vi "加减乘除运算.vi"(1 "符号":string[](array[string]), 2 "元素":string[](array[string])) -> (0 "结果":string)   [LabVIEW 2014]
panel:
  out "输出符号":string[](array[string])
  out "输出元素":string[](array[string])
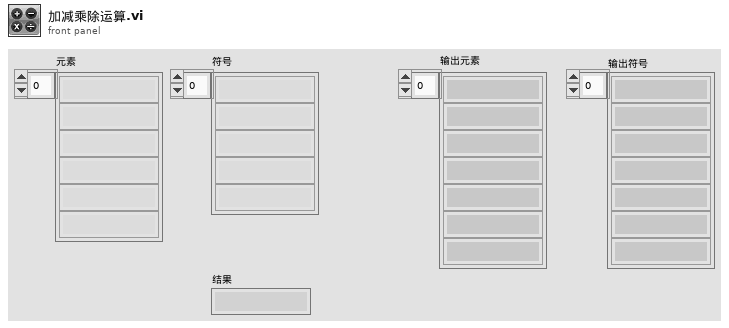
[diagram p1: front panel]
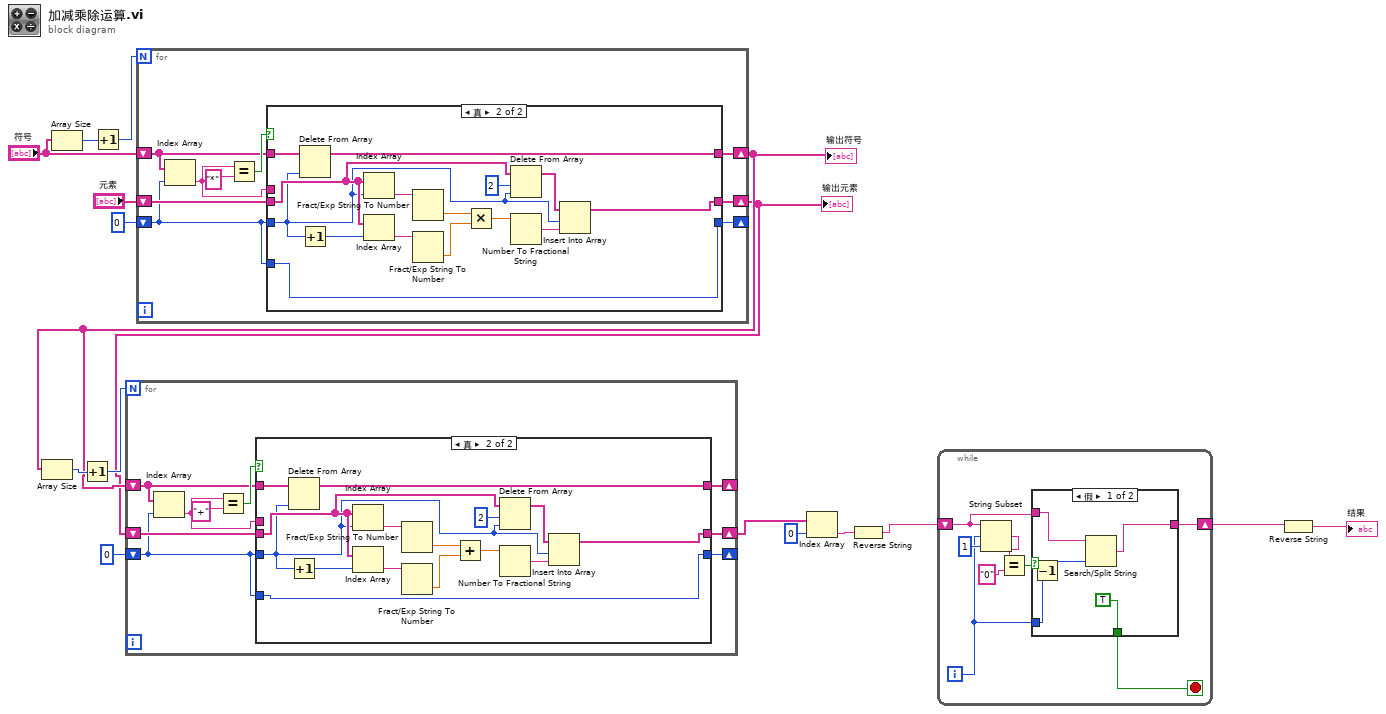
[diagram p0: block diagram]
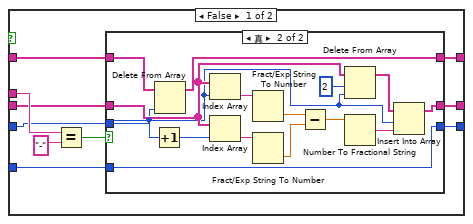
[diagram p3: hidden frame]
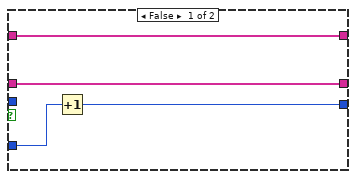
[diagram p4: hidden frame]
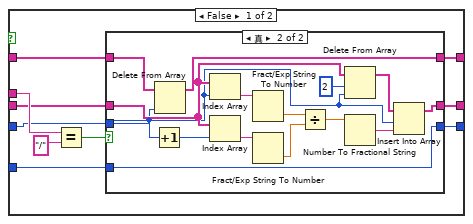
[diagram p5: hidden frame]
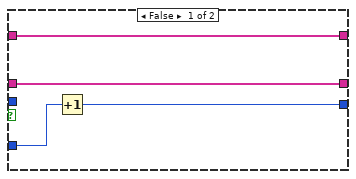
[diagram p6: hidden frame]
diagram:
  n1 = Array Size(array="符号") -> (size(s)=w14:i32)
  n2 = Increment(x=w14) -> (x+1=w13:i32)
  n3 = for {
    N: w13 -> [_]
    shift-right: [w22] -> w7
    shift-left: "元素" -> [w23]
    shift-right: [w19] -> w8
    shift-left: "符号" -> [w20]
    shift-right: [w17] -> _
    shift-left: 0 -> [w18]
    n4 = Index Array(array=w20, index=w18) -> (element=w21:string)
    n5 = Equal?(x=w21, y="*") -> (x = y?=w24:bool)
    n6 = case shown="真" w24 {
      tunnel: w23 -> [w32 w65]
      tunnel: w18 -> [w31 w57]
      tunnel: [w30 w59] -> w22
      tunnel: w21 -> [w34 _]
      tunnel: w20 -> [w29 w58]
      tunnel: [w28 w56] -> w19
      tunnel: w18 -> [w27 w55]
      tunnel: [w26 w55] -> w17
      frame False {
        n7 = Equal?(x=w34, y="/") -> (x = y?=w33:bool)
        n8 = case shown="真" w33 {
          tunnel: w32 -> [w39 w45]
          tunnel: w31 -> [_ w42]
          tunnel: [w39 w44] -> w30
          tunnel: [w38 w41] -> w28
          tunnel: w29 -> [w38 w43]
          tunnel: w27 -> [w37 w40]
          tunnel: [w36 w40] -> w26
          frame False {
            n9 = Increment(x=w37) -> (x+1=w36:i32)
          }
          frame True {
            n10 = Increment(x=w42) -> (x+1=w48:i32)
            n11 = Delete From Array(array=w43, index=w42) -> (array with subset deleted=w41:string[])  [unwired: 1 in, 1 out]
            n12 = Index Array(array=w45, index=w42) -> (element=w54:string)
            n13 = Index Array(array=w45, index=w48) -> (element=w53:string)
            n14 = Fract/Exp String To Number(string=w54) -> (number=w52:dbl)  [unwired: 3 in, 1 out]
            n15 = Fract/Exp String To Number(string=w53) -> (number=w51:dbl)  [unwired: 3 in, 1 out]
            n16 = Divide(x=w52, y=w51) -> (x/y=w47:dbl)
            n17 = Delete From Array(array=w45, length=2 ("长度"), index=w42) -> (array with subset deleted=w49:string[])  [unwired: 1 out]
            n18 = Number To Fractional String(number=w47) -> (F-format string=w46:string)  [unwired: 3 in]
            n19 = Insert Into Array(array=w49, index=w42, new element=w46) -> (w44:string[])
          }
        }
      }
      frame True {
        n20 = Delete From Array(array=w58, index=w57) -> (array with subset deleted=w56:string[])  [unwired: 1 in, 1 out]
        n21 = Increment(x=w57) -> (x+1=w62:i32)
        n22 = Index Array(array=w65, index=w57) -> (element=w69:string)
        n23 = Index Array(array=w65, index=w62) -> (element=w68:string)
        n24 = Fract/Exp String To Number(string=w69) -> (number=w67:dbl)  [unwired: 3 in, 1 out]
        n25 = Fract/Exp String To Number(string=w68) -> (number=w66:dbl)  [unwired: 3 in, 1 out]
        n26 = Multiply(x=w67, y=w66) -> (x*y=w61:dbl)
        n27 = Delete From Array(array=w65, length=2 ("长度"), index=w57) -> (array with subset deleted=w63:string[])  [unwired: 1 out]
        n28 = Number To Fractional String(number=w61) -> (F-format string=w60:string)  [unwired: 3 in]
        n29 = Insert Into Array(array=w63, index=w57, new element=w60) -> (w59:string[])
      }
    }
  }
  "输出元素" <- w7
  "输出符号" <- w8
  n30 = Array Size(array=w8) -> (size(s)=w9:i32)
  n31 = Increment(x=w9) -> (x+1=w10:i32)
  n32 = for {
    N: w10 -> [_]
    shift-right: [w75] -> w6
    shift-left: w7 -> [w76]
    shift-right: [w72] -> _
    shift-left: w8 -> [w73]
    shift-right: [w70] -> _
    shift-left: 0 -> [w71]
    n33 = Index Array(array=w73, index=w71) -> (element=w74:string)
    n34 = Equal?(x=w74, y="+") -> (x = y?=w77:bool)
    n35 = case shown="真" w77 {
      tunnel: w76 -> [w85 w118]
      tunnel: w71 -> [w84 w110]
      tunnel: [w83 w112] -> w75
      tunnel: w74 -> [w87 _]
      tunnel: w73 -> [w82 w111]
      tunnel: [w81 w109] -> w72
      tunnel: w71 -> [w80 w108]
      tunnel: [w79 w108] -> w70
      frame False {
        n36 = Equal?(x=w87, y="-") -> (x = y?=w86:bool)
        n37 = case shown="真" w86 {
          tunnel: w85 -> [w92 w98]
          tunnel: w84 -> [_ w95]
          tunnel: [w92 w97] -> w83
          tunnel: [w91 w94] -> w81
          tunnel: w82 -> [w91 w96]
          tunnel: w80 -> [w90 w93]
          tunnel: [w89 w93] -> w79
          frame False {
            n38 = Increment(x=w90) -> (x+1=w89:i32)
          }
          frame True {
            n39 = Increment(x=w95) -> (x+1=w101:i32)
            n40 = Delete From Array(array=w96, index=w95) -> (array with subset deleted=w94:string[])  [unwired: 1 in, 1 out]
            n41 = Index Array(array=w98, index=w95) -> (element=w107:string)
            n42 = Index Array(array=w98, index=w101) -> (element=w106:string)
            n43 = Fract/Exp String To Number(string=w107) -> (number=w105:dbl)  [unwired: 3 in, 1 out]
            n44 = Fract/Exp String To Number(string=w106) -> (number=w104:dbl)  [unwired: 3 in, 1 out]
            n45 = Subtract(x=w105, y=w104) -> (x-y=w100:dbl)
            n46 = Delete From Array(array=w98, length=2 ("长度"), index=w95) -> (array with subset deleted=w102:string[])  [unwired: 1 out]
            n47 = Number To Fractional String(number=w100) -> (F-format string=w99:string)  [unwired: 3 in]
            n48 = Insert Into Array(array=w102, index=w95, new element=w99) -> (w97:string[])
          }
        }
      }
      frame True {
        n49 = Delete From Array(array=w111, index=w110) -> (array with subset deleted=w109:string[])  [unwired: 1 in, 1 out]
        n50 = Increment(x=w110) -> (x+1=w115:i32)
        n51 = Index Array(array=w118, index=w110) -> (element=w122:string)
        n52 = Index Array(array=w118, index=w115) -> (element=w121:string)
        n53 = Fract/Exp String To Number(string=w122) -> (number=w120:dbl)  [unwired: 3 in, 1 out]
        n54 = Fract/Exp String To Number(string=w121) -> (number=w119:dbl)  [unwired: 3 in, 1 out]
        n55 = Add(x=w120, y=w119) -> (x+y=w114:dbl)
        n56 = Delete From Array(array=w118, length=2 ("长度"), index=w110) -> (array with subset deleted=w116:string[])  [unwired: 1 out]
        n57 = Number To Fractional String(number=w114) -> (F-format string=w113:string)  [unwired: 3 in]
        n58 = Insert Into Array(array=w116, index=w110, new element=w113) -> (w112:string[])
      }
    }
  }
  n59 = Index Array(array=w6, index=0 ("索引")) -> (element=w4:string)
  n60 = Reverse String(1:w4) -> (0:w3:string)
  n61 = while {
    shift-right: [w125] -> w2
    shift-left: w3 -> [w126]
    i -> [w124]
    stop <- w123 stop-if-true
    n62 = String Subset(string=w126, offset (0)=w124, length (rest)=1 ("长度（剩余）")) -> (substring=w128:string)
    n63 = Equal?(x=w128, y="0") -> (x = y?=w129:bool)
    n64 = case shown="假" w129 {
      tunnel: w126 -> [w135 w136]
      tunnel: [w134 w136] -> w125
      tunnel: w124 -> [w132 _]
      tunnel: [TRUE _] -> w123
      frame False {
        n65 = Decrement(x=w132) -> (x-1=w131:i32)
        n66 = Search/Split String(string=w135, offset (0)=w131) -> (match + rest of string=w134:string)  [unwired: 1 in, 2 out]
      }
      frame True {
      }
    }
  }
  n67 = Reverse String(1:w2) -> (0:→"结果":string)
